vi "Get Archive Record Ex V.vi"(8 "error in (no error)":errorcluster, 10 "i":i16, 11 "newRecordStruct":T1) -> (0 "error out":errorcluster, 2 "function return":i16, 3 "newRecordStruct out":T1)   [LabVIEW 2009, in "VantagePro.lvlib"]
doc: "DllAccess short int _stdcall GetArchiveRecordEx_V(WeatherRecordStructEx* newRecordStruct, short int i);"
uses:
  VantagePro.lvlib
  <userlib>/VantagePro/VantagePro.dll
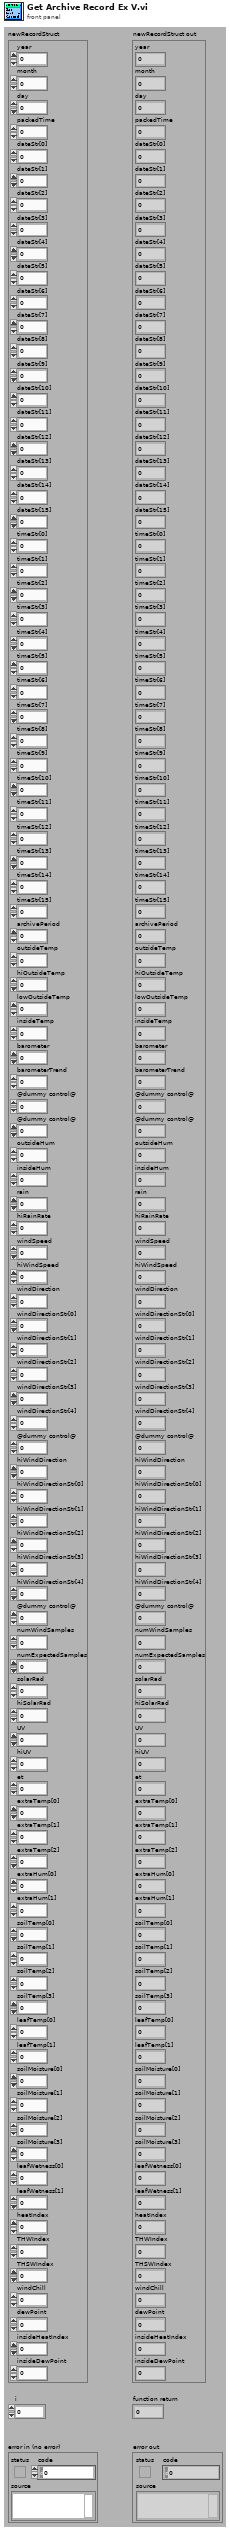
[diagram p1: front panel]
types:
  T1 = cluster{"year":i16, "month":i8, "day":i8, "packedTime":i16, "dateStr[0]":i8, "dateStr[1]":i8, "dateStr[2]":i8, "dateStr[3]":i8, "dateStr[4]":i8, "dateStr[5]":i8, "dateStr[6]":i8, "dateStr[7]":i8, "dateStr[8]":i8, "dateStr[9]":i8, "dateStr[10]":i8, "dateStr[11]":i8, "dateStr[12]":i8, "dateStr[13]":i8, "dateStr[14]":i8, "dateStr[15]":i8, "timeStr[0]":i8, "timeStr[1]":i8, "timeStr[2]":i8, "timeStr[3]":i8, "timeStr[4]":i8, "timeStr[5]":i8, "timeStr[6]":i8, "timeStr[7]":i8, "timeStr[8]":i8, "timeStr[9]":i8, "timeStr[10]":i8, "timeStr[11]":i8, "timeStr[12]":i8, "timeStr[13]":i8, "timeStr[14]":i8, "timeStr[15]":i8, "archivePeriod":i16, "outsideTemp":sgl, "hiOutsideTemp":sgl, "lowOutsideTemp":sgl, "insideTemp":sgl, "barometer":sgl, "barometerTrend":i16, "@dummy control@":i8, "@dummy control@":i8, "outsideHum":sgl, "insideHum":sgl, "rain":sgl, "hiRainRate":sgl, "windSpeed":sgl, "hiWindSpeed":sgl, "windDirection":i16, "windDirectionStr[0]":i8, "windDirectionStr[1]":i8, "windDirectionStr[2]":i8, "windDirectionStr[3]":i8, "windDirectionStr[4]":i8, "@dummy control@":i8, "hiWindDirection":i16, "hiWindDirectionStr[0]":i8, "hiWindDirectionStr[1]":i8, "hiWindDirectionStr[2]":i8, "hiWindDirectionStr[3]":i8, "hiWindDirectionStr[4]":i8, "@dummy control@":i8, "numWindSamples":i16, "numExpectedSamples":i16, "solarRad":i16, "hiSolarRad":i16, "UV":sgl, "hiUV":sgl, "et":sgl, "extraTemp[0]":sgl, "extraTemp[1]":sgl, "extraTemp[2]":sgl, "extraHum[0]":sgl, "extraHum[1]":sgl, "soilTemp[0]":sgl, "soilTemp[1]":sgl, "soilTemp[2]":sgl, "soilTemp[3]":sgl, "leafTemp[0]":sgl, "leafTemp[1]":sgl, "soilMoisture[0]":sgl, "soilMoisture[1]":sgl, "soilMoisture[2]":sgl, "soilMoisture[3]":sgl, "leafWetness[0]":sgl, "leafWetness[1]":sgl, "heatIndex":sgl, "THWIndex":sgl, "THSWIndex":sgl, "windChill":sgl, "dewPoint":sgl, "insideHeatIndex":sgl, "insideDewPoint":sgl}
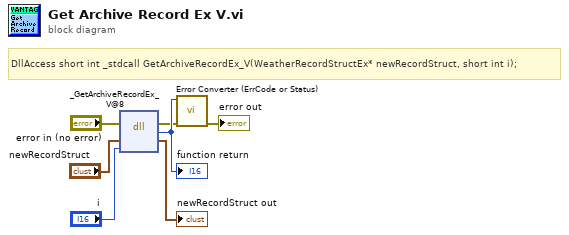
[diagram p0: block diagram]
diagram:
  # "DllAccess short int _stdcall GetArchiveRecordEx_V(WeatherRecordStructEx* newRecordStruct, short int i);"
  n1 = dll-call lib="C:/Program Files/National Instruments/LabVIEW 2010/user.lib/VantagePro/VantagePro.*" fn="_GetArchiveRecordEx_V@8"(error in="error in (no error)", "newRecordStruct"="newRecordStruct", "i"="i") -> (error out=w2:errorcluster, w7:i16, "newRecordStruct"=→"newRecordStruct out":T1)  [unwired: 3 in, 1 out]
  "function return" <- w7
  n2 = call "Error Converter (ErrCode or Status).vi"("error in (no error)"=w2, "error code"=w7) -> ("error out"=→"error out":errorcluster)  [unwired: 9 in]
